vi "AcquisitionDone.vi"(8 "error in (no error)":errorcluster, 10 "Acq Done Data":T1, 11 "Arduino_TranslationStage_UI.lvlib:Arduino_Stepper.lvclass":refnum<class "Arduino_Stepper_UI.lvclass">) -> (0 "error out":errorcluster, 3 "Arduino_TranslationStage_UI.lvlib:Arduino_Stepper.lvclass":refnum<class "Arduino_Stepper_UI.lvclass">)   [LabVIEW 2023, in "Arduino_TranslationStage_UI.lvlib" / "Arduino_Stepper_UI.lvclass"]
uses:
  Arduino_Stepper_UI.lvclass
  Arduino_Stepper_UI.lvclass/Arduino_Stepper_UI.ctl
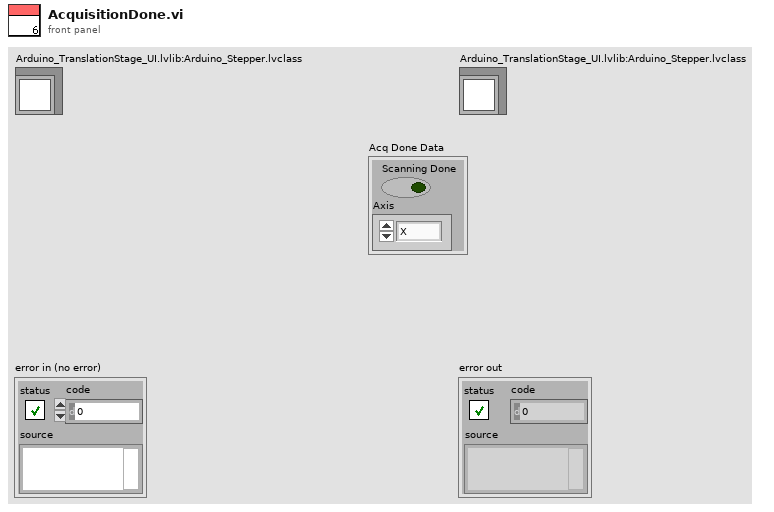
[diagram p1: front panel]
types:
  T1 = cluster{"Scanning Done":bool, "Axis":enum16{"X", "Y", "Z", "HOM"}}
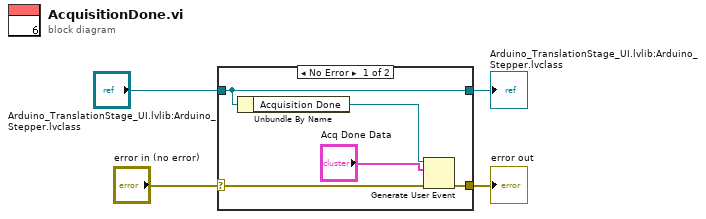
[diagram p0: block diagram]
diagram:
  n1 = case shown="No Error" "error in (no error)" {
    selector: "error in (no error)" -> [w8 w11]
    tunnel: [w7 w11] -> w1
    tunnel: [w6 w10] -> w3
    tunnel: "Arduino_TranslationStage_UI.lvlib:Arduino_Stepper.lvclass" -> [w6 w10]
    frame No Error {
      n2 = Unbundle By Name(w6) -> ("Acquisition Done"=w9:refnum<user-event>)
      n3 = Generate User Event(user event=w9, event data cluster="Acq Done Data", error in=w8) -> (error out=w7:errorcluster)  [unwired: 1 in, 1 out]
    }
    frame Error {
    }
  }
  "error out" <- w1
  "Arduino_TranslationStage_UI.lvlib:Arduino_Stepper.lvclass" <- w3
